vi "reference-generator.vi"(8 "SamplingInt(s)":dbl, 9 "LockinPhase":dbl, 10 "LockinFreq":dbl, 11 "IntegrationPeriod(s)":dbl) -> (3 "output cluster":cluster{dbl[], dbl[]})   [LabVIEW 2013]
doc: "Generates the Lock-In's reference signal."
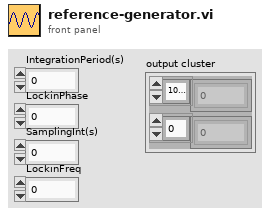
[diagram p1: front panel]
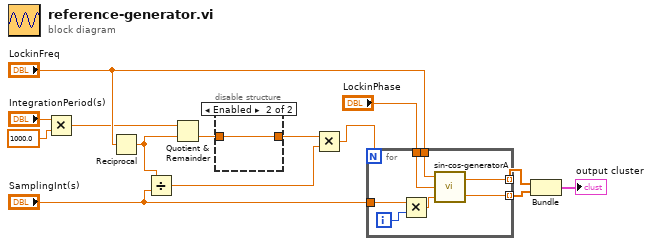
[diagram p0: block diagram]
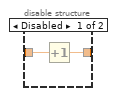
[diagram p2: hidden frame]
diagram:
  n1 = Multiply(x="IntegrationPeriod(s)", y=1000.0) -> (x*y=w2:dbl)
  n2 = Reciprocal(x="LockinFreq") -> (1/x=w5:dbl)
  n3 = Divide(x=w5, y="SamplingInt(s)") -> (x/y=w8:dbl)
  n4 = Quotient & Remainder(x=w2, y=w5) -> (floor(x/y)=w11:dbl)  [unwired: 1 out]
  n5 = disable-structure shown="Enabled" {
    disable-tunnel: w11 -> [w16 w17]
    disable-tunnel: [w15 w17] -> w7
    frame Disabled {
      n6 = Increment(x=w16) -> (x+1=w15:dbl)
    }
    frame Enabled {
    }
  }
  n7 = Multiply(x=w7, y=w8) -> (x*y=w9:dbl)
  n8 = for {
    N: w9 -> [_]
    tunnel: "LockinPhase" -> [w24]
    tunnel: "LockinFreq" -> [w23]
    tunnel: "SamplingInt(s)" -> [w21]
    tunnel: [w19] -> w14 mode=indexing
    tunnel: [w18] -> w13 mode=indexing
    i -> [w22]
    n9 = Multiply(x=w21, y=w22) -> (x*y=w20:dbl)
    n10 = call "sin-cos-generatorA.vi"("Time"=w20, "Phase"=w24, "Frequency"=w23) -> ("cos"=w18:dbl, "sin"=w19:dbl)
  }
  n11 = Bundle(w14, w13) -> (→"output cluster":cluster{dbl[], dbl[]})  [unwired: 1 in]
